vi "Stop Logging.vi"(8 "error in (no error)":errorcluster, 10 "Q":refnum<class "Message Enqueuer.lvclass">, 11 "Classic Logger in":refnum<class "Classic Logger.lvclass">) -> (0 "error out":errorcluster, 3 "Classic Logger out":refnum<class "Classic Logger.lvclass">)   [LabVIEW 2017, in "MGI-Monitored Actor.lvlib" / "Classic Logger.lvclass"]
uses:
  Classic Logger.lvclass
  <vilib>/ActorFramework/Message Enqueuer/Message Enqueuer.lvclass
  Classic Logger.lvclass/Classic Logger.ctl
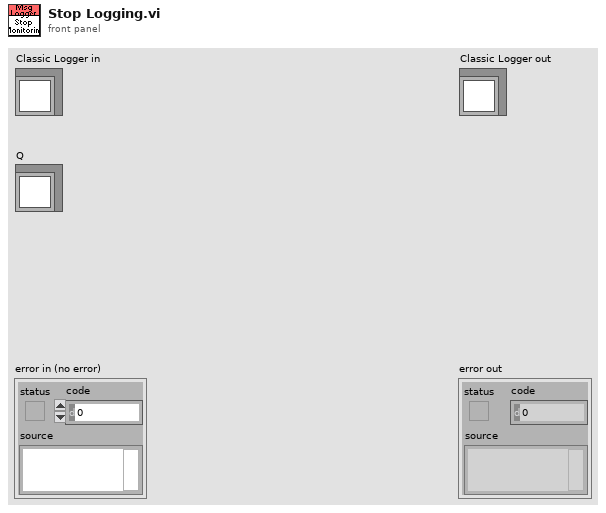
[diagram p1: front panel]
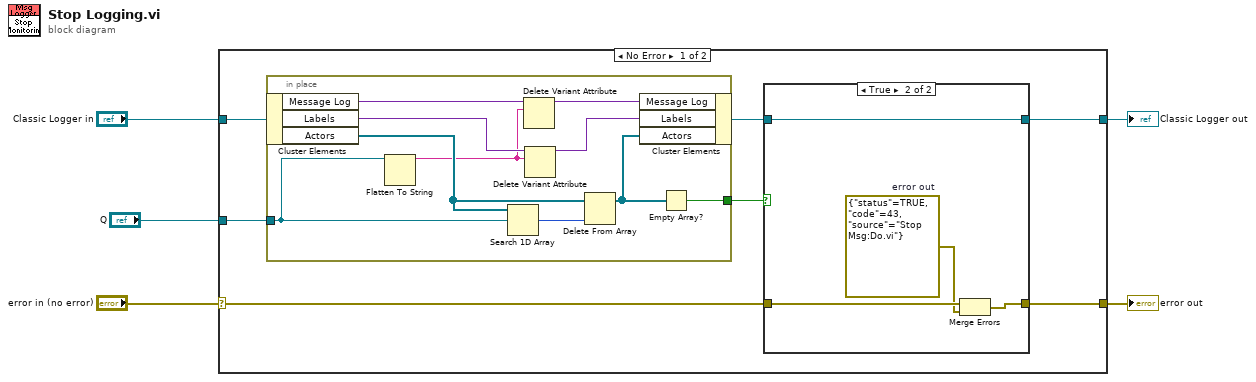
[diagram p0: block diagram]
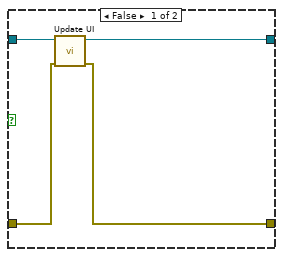
[diagram p2: hidden frame]
diagram:
  n1 = case shown="No Error" "error in (no error)" {
    selector: "error in (no error)" -> [w8 w32]
    tunnel: [w7 w32] -> w4
    tunnel: [w9 w31] -> w2
    tunnel: "Classic Logger in" -> [w11 w31]
    tunnel: "Q" -> [w12 _]
    frame No Error {
      n2 = in-place {
        in-place-border: w12 -> [w28]
        in-place-border: [w21] -> w6
        n3 = in-place-cluster #1(w11) -> ("Message Log"=w25:variant, "Labels"=w27:variant, "Actors"=w29:refnum<class "Message Enqueuer.lvclass">[])
        n4 = Flatten To String(anything=w28) -> (data string=w23:string)  [unwired: 3 in, 2 out]
        n5 = Search 1D Array(1D array=w29, element=w28) -> (index of element=w30:i32)  [unwired: 1 in]
        n6 = Delete Variant Attribute(6:w23, 7:w25) -> (3:w24:variant)  [unwired: 1 in, 2 out]
        n7 = Delete Variant Attribute(6:w23, 7:w27) -> (3:w26:variant)  [unwired: 1 in, 2 out]
        n8 = Delete From Array(array=w29, index=w30) -> (array with subset deleted=w22:refnum<class "Message Enqueuer.lvclass">[])  [unwired: 1 in, 1 out]
        n9 = in-place-cluster #1("Message Log"=w24, "Labels"=w26, "Actors"=w22) -> (w10:refnum<class "Classic Logger.lvclass">)
        n10 = Empty Array?(array=w22) -> (empty?=w21:bool)
      }
      n11 = case shown="True" w6 {
        tunnel: w10 -> [w16 w20]
        tunnel: [w15 w20] -> w9
        tunnel: w8 -> [w14 w19]
        tunnel: [w13 w18] -> w7
        frame False {
          n12 = call "Update UI.vi"("error in (no error)"=w14, "Message Logger in"=w16) -> ("error out"=w13:errorcluster, "Message Logger out"=w15:refnum<class "Classic Logger.lvclass">)  [unwired: 8 in]
        }
        frame True {
          w17 = errorcluster {"status"=TRUE, "code"=43, "source"="Stop Msg:Do.vi"}  # error out
          n13 = Merge Errors(w19, w17) -> (w18:errorcluster)
        }
      }
    }
    frame Error {
    }
  }
  "error out" <- w4
  "Classic Logger out" <- w2
